vi "simple Xcvr (FPGA).vi"() -> ()   [LabVIEW 2021]
doc: "Acquires data from the Rx ports and streams the data to the host while receiving data from the host and generating the resulting waveform at the Tx ports of the NI USRP-294x/295x device. Use this VI as a template for the Simple NI-USRP Streaming sample project."
uses:
  <instrlib>/_niInstr/Register Bus/v1/FPGA/Public/Read Cmd Data.ctl
  <instrlib>/_niInstr/DSP/v1/Shared/Public/IQ Impairments.ctl
  <vilib>/Platform/TimedLoop/XDataNode/timing_clust.ctl
  <vilib>/Platform/TimedLoop/XDataNode/nitl_modes.ctl
  <vilib>/Platform/TimedLoop/XDataNode/wakeup.ctl
  <instrlib>/_niInstr/DSP/v1/Shared/Public/IQ Data.ctl
  <vilib>/rvi/Emulation/niFpgaSctlEmulationGetInTimedLoop.vi
  <vilib>/rvi/Emulation/niFpgaEmulationReportErrorSimple.vi
  <vilib>/rvi/Emulation/niFpgaGetClockAttributes.vi
  <vilib>/rvi/Emulation/niFpgaCriticalErrorInLSC.vi
  <instrlib>/_niInstr/DSP/v1/FPGA/Public/Sub VIs/Frequency Shift/Frequency Shift - 1 spc.vi
  <instrlib>/_niInstr/DSP/v1/FPGA/Public/Sub VIs/IQ Impairments/IQ Impairments - 1 spc.vi
  <instrlib>/_niInstr/DSP/v1/FPGA/Public/Sub VIs/Data Conversion/IQ to I16 - 1 spc - S18.1.vi
  <vilib>/rvi/eio/common/nirviEmuTemplateMethod_errors.vi
  <instrlib>/_niInstr/DSP/v1/FPGA/Public/Sub VIs/Data Conversion/I16 to IQ - 1 spc - S18.1.vi
  <instrlib>/_niInstr/DSP/v1/FPGA/Public/Sub VIs/Data Conversion/IQ to U32 - 1 spc - S18.1.vi
  <vilib>/rvi/interface/RandomDataEmulation/niFpgaRandomDataHandleErrors.vi
  <vilib>/Platform/TimedLoop/XDataNode/XDataNode.xnode
  <vilib>/eio/EIONode/EIONode.xnode
  <vilib>/rvi/DataTransferAndStorage/Container/XNode/niFpgaContainer.xnode
  <vilib>/rvi/interface/RandomDataEmulation/nirviRandomDataFpgaReadWriteTemplate.vi
  <vilib>/Platform/TimedLoop/XDataNode/XDNodeRunTimeDep.lvlib
  <instrlib>/_niInstr/Register Bus/v1/FPGA/niInstr Register Bus v1 FPGA.lvlib
  <instrlib>/niUsrpRio/Config/v1/FPGA/niUsrpRio Config v1 FPGA.lvlib
  <instrlib>/_niInstr/DSP/v1/FPGA/niInstr DSP v1 FPGA.lvlib
  <instrlib>/_niInstr/DSP/v1/Shared/niInstr DSP v1 Shared.lvlib
panel:
  in  "send data to host":bool[](array[boolean])=[FALSE, FALSE]
  in  "Tx params":T1(array[cluster])=[{"linear amp"=0.0, "frequency shift"=0.0}, {"linear amp"=0.0, "frequency shift"=0.0}] {"frequency shift" format="%#.48g"}
  in  "DDC params":T2(array[cluster])=[{"frequency shift"=0.0, "output sample rate"=0.0}, {"frequency shift"=0.0, "output sample rate"=0.0}] {"output sample rate" format="%.48g"; "frequency shift" format="%#.48g"}
  in  "impairments":T3[](array[typedef])
  in  "reset":bool
  in  "start trigger":bool
  in  "rx 3.led":T4(ring)
  in  "rx 2.led":T4(ring)
  in  "rx 0.led":T4(ring)
  in  "rx 1.led":T4(ring)
  in  "tx 0.led":enum16{"None", "RF 0/TX 1", "RF 1/TX 1"}(ring)
  in  "tx 1.led":enum16{"None", "RF 0/TX 1", "RF 1/TX 1"}(ring)
  in  "rx 3.stream enable":bool
  in  "rx 2.stream enable":bool
  out "rx 3.number of iq data overflows":u64
  out "rx 2.number of iq data overflows":u64
  in  "rx 3.phase":fxp<+/-,21,0>
  in  "rx 3.frequency shift":fxp<+/-,48,0> format="%#.48g"
  in  "rx 3.impairments":T3={"inline gain I"=0.9999923706054688, "inline gain Q"=0.9999923706054688, "cross gain I"=0.0, "cross gain Q"=0.0, "pre-gain offset I"=0.0, "pre-gain offset Q"=0.0, "post-gain offset I"=0.0, "post-gain offset Q"=0.0}
  in  "rx 2.phase":fxp<+/-,21,0>
  in  "rx 2.frequency shift":fxp<+/-,48,0> format="%#.48g"
  in  "rx 2.impairments":T3={"inline gain I"=0.9999923706054688, "inline gain Q"=0.9999923706054688, "cross gain I"=0.0, "cross gain Q"=0.0, "pre-gain offset I"=0.0, "pre-gain offset Q"=0.0, "post-gain offset I"=0.0, "post-gain offset Q"=0.0}
  in  "RF 1/Tx/Enable":bool
  in  "RF 1/Rx/Enable":bool
  in  "RF 0/Tx/Enable":bool
  in  "RF 0/Rx/Enable":bool
  in  "reg.host read.go rcvd 0":bool
  out "reg.notify host.go 0":bool
  in  "reg.notify host.go rcvd 0":bool
  out "reg.host read.data 0":T5
  in  "reg.reset 0":bool
  # "FPGA utilization for 200 MS/s"
  # "FPGA utilization for 120 MS/s"
  # "USRP RIO Simple Streaming FPGA"
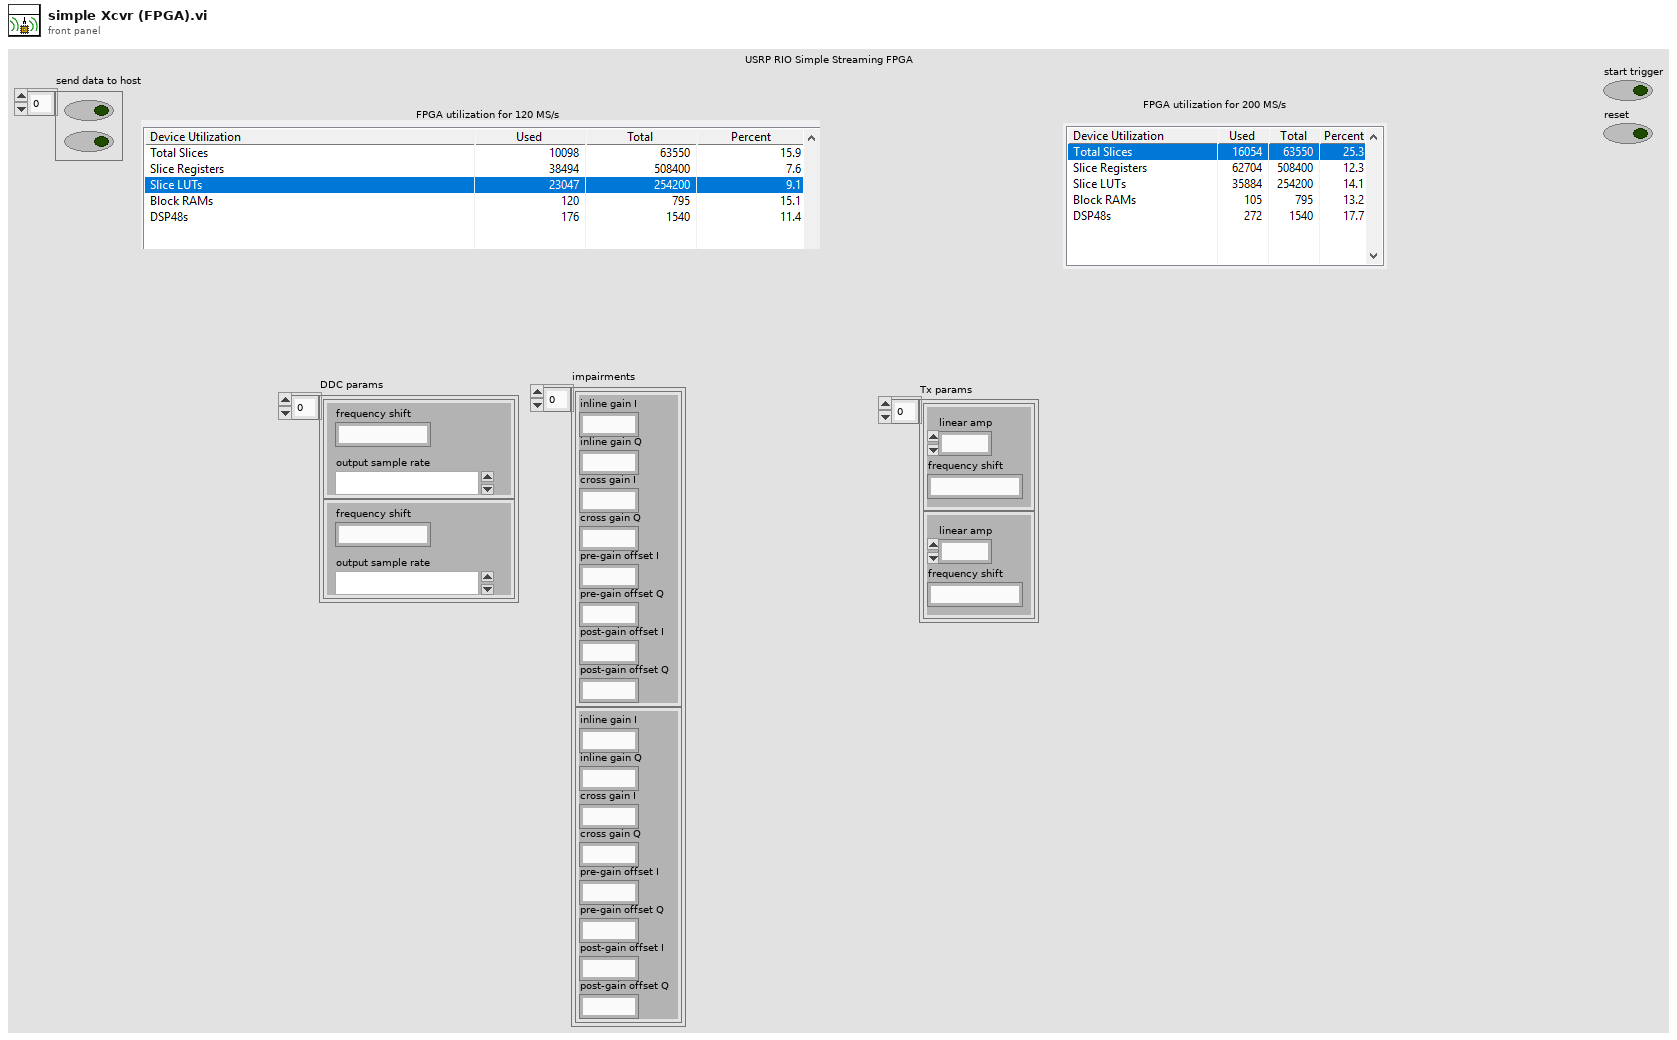
[diagram p1: front panel]
types:
  T1 = cluster{"linear amp":fxp<+/-,18,1>, "frequency shift":fxp<+/-,48,0>}[]
  T2 = cluster{"frequency shift":fxp<+/-,48,0>, "output sample rate":fxp<+,48,1>}[]
  T3 = typedef "niInstr DSP v1 Shared.lvlib/IQ Impairments.ctl" = cluster{"inline gain I":fxp<+/-,18,1>, "inline gain Q":fxp<+/-,18,1>, "cross gain I":fxp<+/-,18,1>, "cross gain Q":fxp<+/-,18,1>, "pre-gain offset I":fxp<+/-,18,1>, "pre-gain offset Q":fxp<+/-,18,1>, "post-gain offset I":fxp<+/-,18,1>, "post-gain offset Q":fxp<+/-,18,1>}
  T4 = enum16{"None", "RF 0/RX 1", "RF 0/RX 2", "RF 1/RX 1", "RF 1/RX 2"}
  T5 = typedef "niInstr Register Bus v1 FPGA.lvlib/Read Cmd Data.ctl" = cluster{"go":bool, "data":u32}
  T6 = typedef "XDNodeRunTimeDep.lvlib/timing_clust.ctl" = cluster{"Expected End [f-1]":u64, "Actual End [f-1]":u64, "Finished Late? [f-1]":bool, "Expected End [i-1]":u64, "Actual End [i-1]":u64, "Finished Late? [i-1]":bool, "Expected Start [i]":u64, "Actual Start [i]":u64, "Expected Start [f]":u64, "Actual Start [f]":u64, "Source Name":string, "Structure Name":string, "Period":i64, "Deadline":i64, "Offset":i64, "Start":i64, "Priority":i32, "Timeout":i32, "Mode":T7, "Wakeup Reason":T8, "Error":errorcluster, "Source Type":string, "Secondary Source Type":string, "Global End Time":u64, "Global Start Time":u64, "Frame Duration":u64, "Iteration Duration":u64, "Assigned CPU":i32, "I/O Scan Engine Mode":u32}
  T7 = typedef "XDNodeRunTimeDep.lvlib/nitl_modes.ctl" = enum32{"No Change", "Process missed periods, maintain original phase", "Discard missed periods, maintain original phase", "Process missed periods, ignore original phase", "Discard missed periods, ignore original phase"}
  T8 = typedef "XDNodeRunTimeDep.lvlib/wakeup.ctl" = enum32{"Normal", "Aborted", "Asynchronous wakeup", "Timing source error", "Timed loop error", "Timeout"}
  T9 = cluster{"tx 0.led":enum16{"None", "RF 0/TX 1", "RF 1/TX 1"}, "tx 1.led ":enum16{"None", "RF 0/TX 1", "RF 1/TX 1"}}
  T10 = cluster{"rx 0.led":enum16{"None", "RF 0/RX 1", "RF 0/RX 2", "RF 1/RX 1", "RF 1/RX 2"}, "rx 1.led":enum16{"None", "RF 0/RX 1", "RF 0/RX 2", "RF 1/RX 1", "RF 1/RX 2"}}
  T11 = cluster{"DAC FIFO Reset":refnum<k21>, "RF 0 Rx Swap IQ":refnum<k21>, "RF 0 Rx Negate I":refnum<k21>, "RF 0 Rx Negate Q":refnum<k21>, "RF 0 Rx Data Valid":refnum<k21>, "RF 0 Rx Data Ever Invalid":refnum<k21>, "clear RF 0 Rx Data Ever Invalid":refnum<k21>, "RF 0 Tx Swap IQ":refnum<k21>, "RF 0 Tx Negate I":refnum<k21>, "RF 0 Tx Negate Q":refnum<k21>, "RF 1 Rx Swap IQ":refnum<k21>, "RF 1 Rx Negate I":refnum<k21>, "RF 1 Rx Negate Q":refnum<k21>, "RF 1 Rx Data Valid":refnum<k21>, "RF 1 Rx Data Ever Invalid":refnum<k21>, "clear RF 1 Rx Data Ever Invalid":refnum<k21>, "RF 1 Tx Swap IQ":refnum<k21>, "RF 1 Tx Negate I":refnum<k21>, "RF 1 Tx Negate Q":refnum<k21>}
  T12 = typedef "niUsrpRio Synchronization v1 FPGA.lvlib/Resources.ctl" = cluster{"master":refnum<k21>, "meas.enable":refnum<k21>, "meas.ready":refnum<k21>, "meas.reset":refnum<k21>, "meas.arm":refnum<k21>, "meas.valid":refnum<k21>, "meas.value":refnum<k21>, "meas.oversample factor":refnum<k21>, "cptr":refnum<k21>, "cptr.adjust":refnum<k21>, "cptr.period":refnum<k21>}
  T13 = typedef "niUsrpRio Time v1 FPGA.lvlib/Time Resources.ctl" = cluster{"reset":refnum<k21>, "time":refnum<k21>, "time.previous cptr":refnum<k21>, "new time":refnum<k21>, "new time.when":refnum<k21>, "new time.set":refnum<k21>, "which edge of ref":refnum<k21>, "pps source":refnum<k21>, "internal pps period":refnum<k21>}
  T14 = typedef "niUsrpRio Time v1 FPGA.lvlib/Future Event Resources.ctl" = cluster{"reset":refnum<k21>, "future event.time":refnum<k21>, "future event.ready":refnum<k21>, "future event.set":refnum<k21>, "future event.clear":refnum<k21>, "future event.set in past":refnum<k21>}
  T15 = cluster{"time.resources":T13, "future event.resources":T14, "future event.resources":T14, "future event.resources":T14}
  T16 = typedef "niInstr Register Bus v1 FPGA.lvlib/Register Instruction.ctl" = cluster{"subsystem":u8, "address":u16, "data":u32, "valid":bool, "read":bool}
  T17 = typedef "niInstr Register Bus v1 FPGA.lvlib/Read Completion.ctl" = cluster{"data":u32, "valid":bool}
  T18 = typedef "niInstr DSP v1 Shared.lvlib/IQ Data.ctl" = cluster{"I":fxp<+/-,18,1>, "Q":fxp<+/-,18,1>, "overflow":bool}
  T19 = cluster{"linear amp":fxp<+/-,18,1>, "frequency shift":fxp<+/-,48,0>}
  T20 = cluster{"frequency shift":fxp<+/-,48,0>, "output sample rate":fxp<+,48,1>}
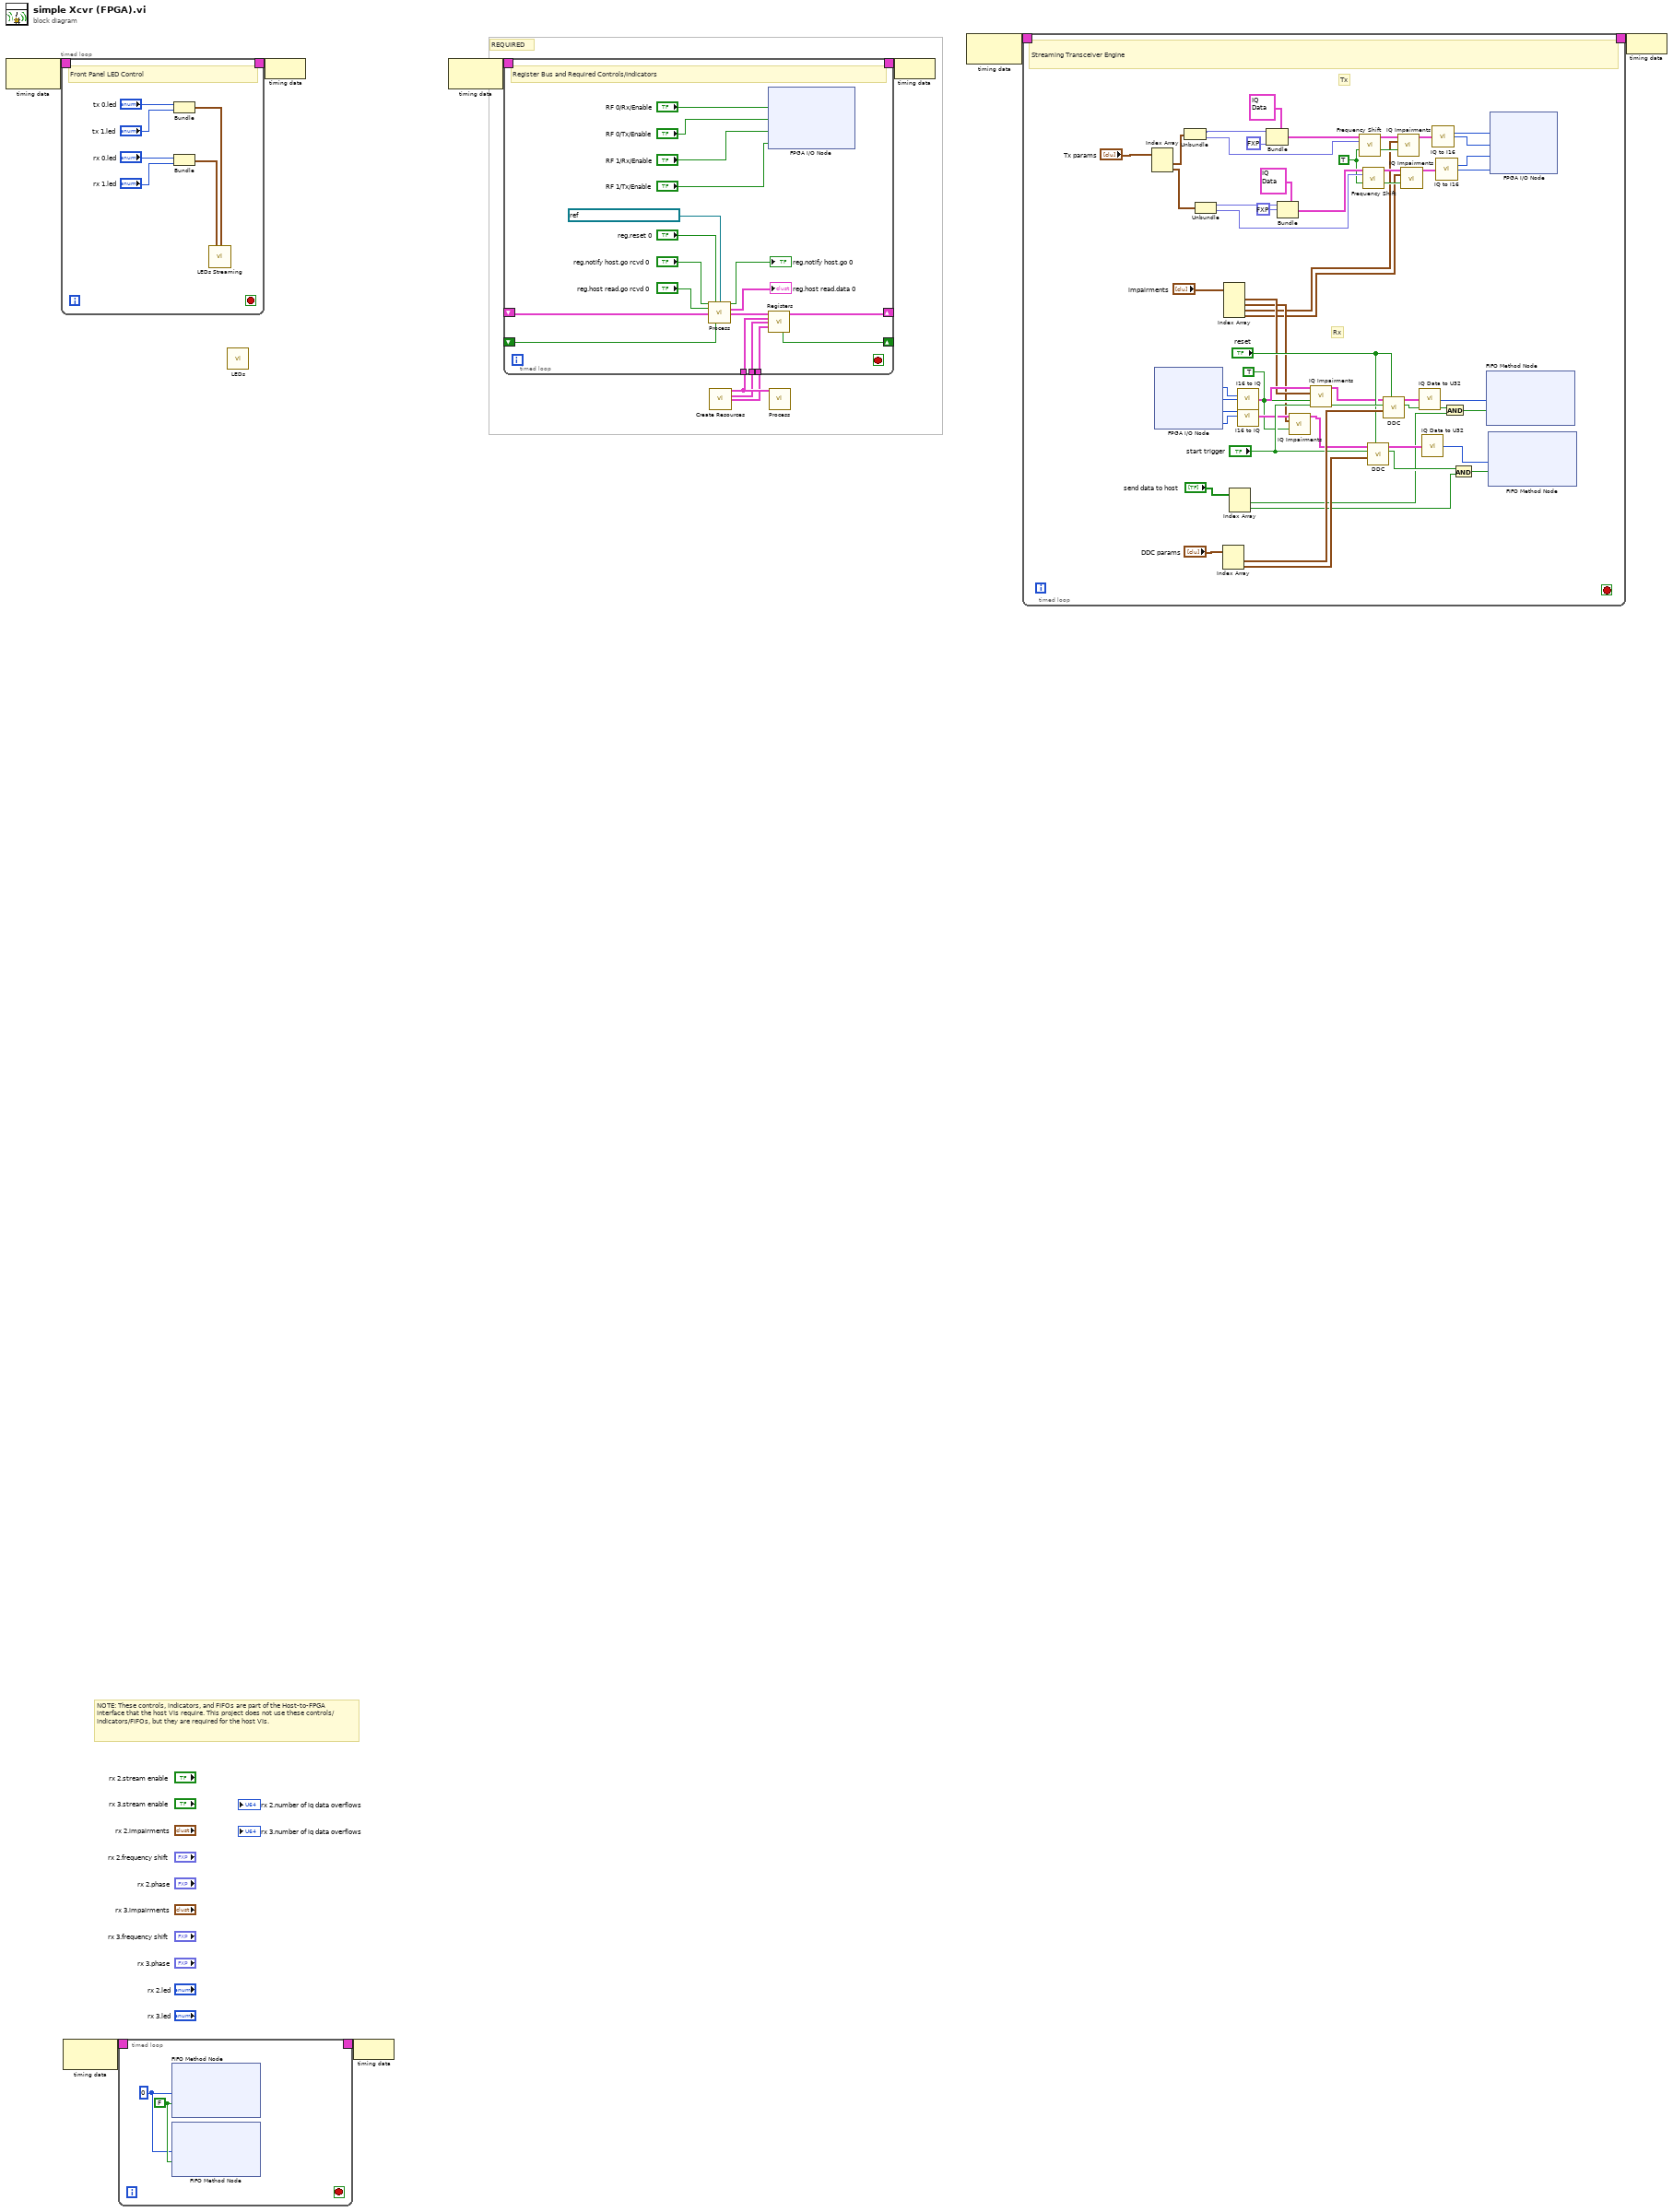
[diagram p0: block diagram]
diagram:
  # "NOTE: These controls, indicators, and FIFOs are part of the Host-to-FPGA interface that the host VIs require. This project does not use these controls/indicators/FIFOs, but they are required for the host VIs."
  # "REQUIRED"
  n1 = node-c288() -> (w2:T6)  [unwired: 1 in]
  n2 = timed-loop {
    timing: w2 -> [_]
    timing-out: [_] -> w1
    stop <- _ stop-if-true
    # "Front Panel LED Control"
    n3 = Bundle("tx 0.led"="tx 0.led", "tx 1.led"="tx 1.led") -> (w12:T9)  [unwired: 1 in]
    n4 = Bundle("rx 0.led"="rx 0.led", "rx 1.led"="rx 1.led") -> (w13:T10)  [unwired: 1 in]
    n5 = call "LEDs Streaming.vi"("rx.leds"=w13, "tx.leds"=w12) -> ()  [unwired: 14 in]
  }
  n6 = node-c288() -> (w4:T6)  [unwired: 1 in]
  n7 = timed-loop {
    timing: w4 -> [_]
    timing-out: [_] -> w3
    stop <- _ stop-if-true
    w20 = u32 0 ("Element")
    w21 = FALSE ("Input Valid")
    n8 = xnode ("FIFO Method Node")("Element"=w20, "Input Valid"=w21) -> ()  [unwired: 1 in, 2 out]
    n9 = xnode ("FIFO Method Node")("Element"=w20, "Input Valid"=w21) -> ()  [unwired: 1 in, 2 out]
  }
  n10 = call "LEDs.vi"() -> ()  [unwired: 1 in]
  n11 = node-c288(w1) -> ()
  n12 = node-c288(w3) -> ()
  n13 = node-c288() -> (w11:T6)  [unwired: 1 in]
  n14 = call "Create Resources.vi"() -> ("config.resources"=w7:T11, "sync.resources"=w6:T12, "time.resources"=w5:T15)  [unwired: 13 in]
  n15 = timed-loop "Register Bus and Required Controls/Indicators" {
    timing: w11 -> [_]
    timing-out: [_] -> w10
    shift-right: [w38] -> _
    shift-left: _ -> [w37]
    shift-right: [w32] -> _
    shift-left: _ -> [w36]
    tunnel: w7 -> [w30]
    tunnel: w6 -> [w29]
    tunnel: w5 -> [w28]
    stop <- _ stop-if-true
    # "Register Bus and Required Controls/Indicators"
    n16 = call <instrlib>:"Process.vi"("reg.notify host.go rcvd"="reg.notify host.go rcvd 0", "reg.reset"="reg.reset 0", "reg.host instruction fifo"=refnum<k21> "reg.host instruction fifo 0", "reg.host read.go rcvd"="reg.host read.go rcvd 0", "read completion"=w37, "ready for output"=w36) -> ("reg.notify host.go"=→"reg.notify host.go 0":bool, "reg.host read.data"=→"reg.host read.data 0":T5, "register instruction"=w31:T16)  [unwired: 7 in]
    n17 = xnode ("FPGA I/O Node")("RF 0/Rx/Enable"="RF 0/Rx/Enable", "RF 0/Tx/Enable"="RF 0/Tx/Enable", "RF 1/Rx/Enable"="RF 1/Rx/Enable", "RF 1/Tx/Enable"="RF 1/Tx/Enable") -> ()  [unwired: 4 in, 4 out]
    n18 = call "Registers.vi"("register instruction"=w31, "config.resources"=w30, "sync.resources"=w29, "time.resources"=w28) -> ("read completion out"=w38:T17, "ready for input"=w32:bool)  [unwired: 10 in]
  }
  n19 = call <instrlib>:"Process.vi"("resources"=w7) -> ()  [unwired: 15 in]
  n20 = node-c288(w10) -> ()
  n21 = node-c288() -> (w9:T6)  [unwired: 1 in]
  n22 = timed-loop "Streaming Transceiver Engine" {
    timing: w9 -> [_]
    timing-out: [_] -> w8
    stop <- _ stop-if-true
    w55 = TRUE ("input valid")
    w86 = TRUE ("input valid")
    # "Rx"
    # "Tx"
    # "Streaming Transceiver Engine"
    n23 = Index Array(array="Tx params") -> (element #1=w63:T19, element #2=w54:T19)  [unwired: 2 in]
    n24 = xnode "FPGA I/O Node"() -> ("RF 0/Rx/I"=w94:i16, "RF 0/Rx/Q"=w95:i16, "RF 1/Rx/I"=w96:i16, "RF 1/Rx/Q"=w97:i16)  [unwired: 4 in, 4 out]
    n25 = Unbundle(w63) -> ("linear amp"=w62:fxp<+/-,18,1>, "frequency shift"=w61:fxp<+/-,48,0>)
    n26 = Unbundle(w54) -> ("linear amp"=w60:fxp<+/-,18,1>, "frequency shift"=w56:fxp<+/-,48,0>)
    n27 = Index Array(array="DDC params") -> (element #1=w93:T20, element #2=w82:T20)  [unwired: 2 in]
    n28 = Index Array(array="impairments") -> (element #1=w84:T3, element #2=w53:T3, element #3=w52:T3, element #4=w51:T3)  [unwired: 4 in]
    n29 = Index Array(array="send data to host") -> (element #1=w45:bool, element #2=w44:bool)  [unwired: 2 in]
    n30 = call-poly <instrlib>:"I16 to IQ.vi"("I"=w94, "Q"=w95) -> ("IQ"=w90:T18)  [unwired: 13 in]
    n31 = call-poly <instrlib>:"I16 to IQ.vi"("I"=w96, "Q"=w97) -> ("IQ"=w88:T18)  [unwired: 13 in]
    n32 = Bundle(cluster=T18 {"I"=0.9999923706054688, "Q"=0.0, "overflow"=FALSE} ("data in"), "I"=w62, "Q"=fxp<+/-,18,1> 0.0) -> (w65:T18)  [unwired: 1 in]
    n33 = Bundle(cluster=T18 {"I"=0.9999923706054688, "Q"=0.0, "overflow"=FALSE} ("data in"), "I"=w60, "Q"=fxp<+/-,18,1> 0.0) -> (w57:T18)  [unwired: 1 in]
    n34 = call-poly <instrlib>:"IQ Impairments.vi"("data in"=w88, "impairments"=w53, "input valid"=w86) -> ("data out"=w87:T18)  [unwired: 9 in, 3 out]
    n35 = call-poly <instrlib>:"IQ Impairments.vi"("data in"=w90, "impairments"=w84, "input valid"=w86) -> ("data out"=w89:T18)  [unwired: 9 in, 3 out]
    n36 = call-poly <instrlib>:"Frequency Shift.vi"("data in"=w65, "frequency shift"=w61, "input valid"=w55) -> ("data out"=w77:T18, "output valid"=w76:bool)  [unwired: 9 in, 2 out]
    n37 = call-poly <instrlib>:"Frequency Shift.vi"("data in"=w57, "frequency shift"=w56, "input valid"=w55) -> ("data out"=w70:T18, "output valid"=w71:bool)  [unwired: 9 in, 2 out]
    n38 = call "DDC.vi"("reset"="reset", "DDC params"=w82, ">> rx start trigger >>"="start trigger", "IQ"=w87) -> ("output valid"=w50:bool, "data out"=w79:T18)  [unwired: 6 in]
    n39 = call "DDC.vi"("reset"="reset", "DDC params"=w93, ">> rx start trigger >>"="start trigger", "IQ"=w89) -> ("output valid"=w48:bool, "data out"=w81:T18)  [unwired: 6 in]
    n40 = call-poly <instrlib>:"IQ Impairments.vi"("data in"=w77, "impairments"=w52, "input valid"=w76) -> ("data out"=w75:T18)  [unwired: 9 in, 3 out]
    n41 = call-poly <instrlib>:"IQ Impairments.vi"("data in"=w70, "impairments"=w51, "input valid"=w71) -> ("data out"=w72:T18)  [unwired: 9 in, 3 out]
    n42 = call-poly <instrlib>:"IQ Data to U32.vi"("IQ data"=w81) -> ("U32 data"=w80:u32)  [unwired: 13 in, 1 out]
    n43 = call-poly <instrlib>:"IQ Data to U32.vi"("IQ data"=w79) -> ("U32 data"=w78:u32)  [unwired: 13 in, 1 out]
    n44 = call-poly <instrlib>:"IQ to I16.vi"("IQ"=w75) -> ("I"=w74:i16, "Q"=w73:i16)  [unwired: 12 in, 1 out]
    n45 = call-poly <instrlib>:"IQ to I16.vi"("IQ"=w72) -> ("I"=w69:i16, "Q"=w68:i16)  [unwired: 12 in, 1 out]
    n46 = And(x=w48, y=w45) -> (x .and. y?=w47:bool)
    n47 = And(x=w50, y=w44) -> (x .and. y?=w49:bool)
    n48 = xnode ("FIFO Method Node")("Element"=w80, "Input Valid"=w47) -> ()  [unwired: 1 in, 2 out]
    n49 = xnode ("FIFO Method Node")("Element"=w78, "Input Valid"=w49) -> ()  [unwired: 1 in, 2 out]
    n50 = xnode "FPGA I/O Node"("RF 0/Tx/I"=w74, "RF 0/Tx/Q"=w73, "RF 1/Tx/I"=w69, "RF 1/Tx/Q"=w68) -> ()  [unwired: 4 in, 4 out]
  }
  n51 = node-c288(w8) -> ()
